vi "Simple cDAQ thermocouple with data logging and timed loop example.vi"() -> ()   [LabVIEW 2015]
uses:
  <vilib>/Platform/TimedLoop/XDataNode/timing_clust.ctl
  <vilib>/Platform/TimedLoop/XDataNode/nitl_modes.ctl
  <vilib>/Platform/TimedLoop/XDataNode/wakeup.ctl
  <vilib>/express/express shared/transition.llb/Dynamic To Waveform Array.vi
  <vilib>/express/express signal manip/GetorSetDDTAttributes/Set DDT Attributes/SetT0.vi
  <vilib>/express/express shared/transition.llb/Waveform Array To Dynamic.vi
  <vilib>/platform/TimedLoop/XDataNode/XDataNode.xnode
  <vilib>/express/express signal manip/GetorSetDDTAttributes/Set DDT Attributes/Set DDT Properties.xnode
  <vilib>/Platform/TimedLoop/XDataNode/XDNodeRunTimeDep.lvlib
panel:
  out "Stop loops":bool
  in  "stop":bool
  out "Temperature":dbl(graph)
  out "Loop counter":i32
  out "Temperature":dbl
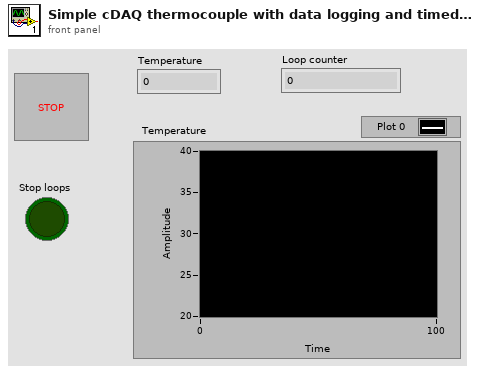
[diagram p1: front panel]
types:
  T1 = typedef "XDNodeRunTimeDep.lvlib/timing_clust.ctl" = cluster{"Expected End [f-1]":u64, "Actual End [f-1]":u64, "Finished Late? [f-1]":bool, "Expected End [i-1]":u64, "Actual End [i-1]":u64, "Finished Late? [i-1]":bool, "Expected Start [i]":u64, "Actual Start [i]":u64, "Expected Start [f]":u64, "Actual Start [f]":u64, "Source Name":string, "Structure Name":string, "Period":i64, "Deadline":i64, "Offset":i64, "Start":i64, "Priority":i32, "Timeout":i32, "Mode":T2, "Wakeup Reason":T3, "Error":errorcluster, "Source Type":string, "Secondary Source Type":string, "Global End Time":u64, "Global Start Time":u64, "Frame Duration":u64, "Iteration Duration":u64, "Assigned CPU":i32, "I/O Scan Engine Mode":u32}
  T2 = typedef "XDNodeRunTimeDep.lvlib/nitl_modes.ctl" = enum32{"No Change", "Process missed periods, maintain original phase", "Discard missed periods, maintain original phase", "Process missed periods, ignore original phase", "Discard missed periods, ignore original phase"}
  T3 = typedef "XDNodeRunTimeDep.lvlib/wakeup.ctl" = enum32{"Normal", "Aborted", "Asynchronous wakeup", "Timing source error", "Timed loop error", "Timeout"}
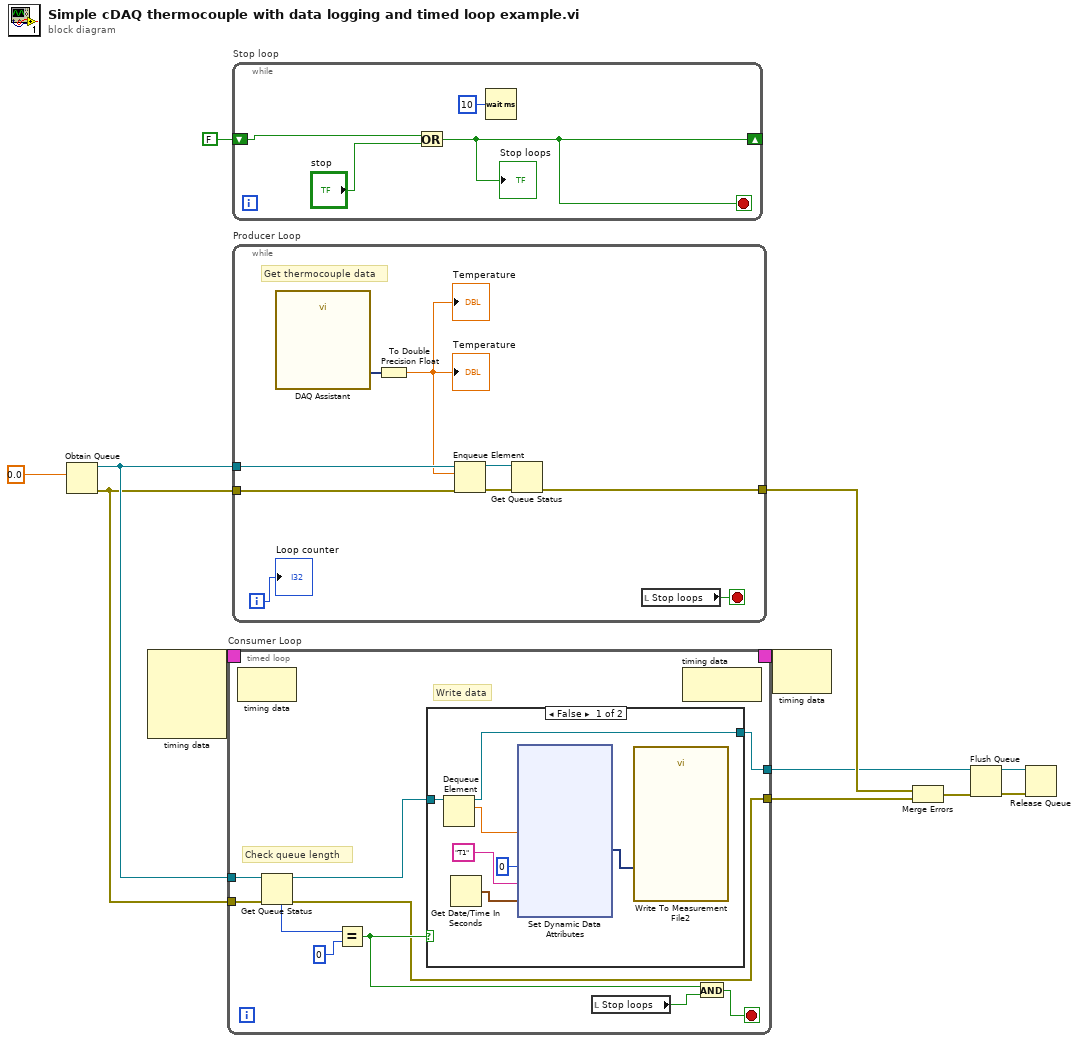
[diagram p0: block diagram]
diagram:
  n1 = Obtain Queue(element data type=0.0) -> (queue out=w4:refnum<queue>, error out=w3:errorcluster)  [unwired: 4 in, 1 out]
  n2 = node-c288() -> (w6:T1)  [unwired: 4 in]
  n3 = timed-loop "Consumer Loop" {
    timing: w6 -> [_]
    timing-out: [_] -> w5
    tunnel: w4 -> [w17]
    tunnel: w3 -> [w16]
    tunnel: [w15] -> w2
    tunnel: [w14] -> w1
    stop <- w13 stop-if-true
    # "Write data"
    # "Check queue length"
    n4 = node-c288() -> ()  [unwired: 1 in, 1 out]
    n5 = Get Queue Status(queue=w17, error in (no error)=w16) -> (queue out=w18:refnum<queue>, error out=w15:errorcluster, # elements in queue=w22:i32)  [unwired: 1 in, 5 out]
    n6 = Equal?(x=w22, y=0) -> (x = y?=w19:bool)
    n7 = case shown="False" w19 {
      tunnel: w18 -> [w24 w47]
      tunnel: [w23 w47] -> w14
      frame False {
        n8 = Dequeue Element(queue=w24) -> (queue out=w23:refnum<queue>, element=w25:dbl)  [unwired: 2 in, 2 out]
        n9 = Get Date/Time In Seconds() -> (seconds since 1Jan1904=w28:timestamp)
        n10 = xnode "Set Dynamic Data Attributes"("Signals In"=w25, "Signal Index"=0, "Signal Name"="T1", "Timestamp"=w28) -> ("Signals Out"=w27:dynamicdata)  [unwired: 1 in, 1 out]
        n11 = call "Write To Measurement File2"("Signals"=w27) -> ()  [unwired: 16 in, 3 out]
      }
      frame True {
      }
    }
    n12 = local read "Stop loops"() -> (w20:bool)
    n13 = node-c288() -> ()  [unwired: 1 in, 1 out]
    n14 = And(x=w19, y=w20) -> (x .and. y?=w13:bool)
  }
  n15 = while "Stop loop" {
    shift-right: [w51] -> _
    shift-left: FALSE -> [w52]
    stop <- w51 stop-if-true
    n16 = Or(x=w52, y="stop") -> (x .or. y?=w51:bool)
    "Stop loops" <- w51
    n17 = Wait (ms)(milliseconds to wait=u32 10) -> ()  [unwired: 1 out]
  }
  n18 = while "Producer Loop" {
    tunnel: w4 -> [w60]
    tunnel: w3 -> [w56]
    tunnel: [w54] -> w9
    i -> [w62]
    stop <- w57 stop-if-true
    # "Get thermocouple data"
    n19 = call "DAQ Assistant"() -> ("data"=w61:dynamicdata)  [unwired: 16 in, 3 out]
    n20 = To Double Precision Float(number=w61) -> (double precision float=w59:dbl)
    "Temperature" <- w59
    "Temperature" <- w59
    n21 = Enqueue Element(queue=w60, element=w59, error in (no error)=w56) -> (queue out=w58:refnum<queue>, error out=w55:errorcluster)  [unwired: 1 in, 1 out]
    n22 = Get Queue Status(queue=w58, error in (no error)=w55) -> (error out=w54:errorcluster)  [unwired: 1 in, 7 out]
    n23 = local read "Stop loops"() -> (w57:bool)
    "Loop counter" <- w62
  }
  n24 = node-c288(w5) -> ()  [unwired: 1 out]
  n25 = Merge Errors(w9, w2) -> (w8:errorcluster)
  n26 = Flush Queue(queue=w1, error in (no error)=w8) -> (queue out=w10:refnum<queue>, error out=w7:errorcluster)  [unwired: 1 out]
  n27 = Release Queue(queue=w10, error in (no error)=w7) -> ()  [unwired: 1 in, 3 out]
